vi "Save File Create Default File.vi"(7 "Type":enum16{"Pass Default", "Write Default"}(ring), 11 "Config Path":path) -> (3 "Default Configuration":string[][](array[string]))   [LabVIEW 2016, in "File Setup.lvlib"]
uses:
  File Setup.lvlib
  <vilib>/Utility/file.llb/Write To Spreadsheet File (string).vi
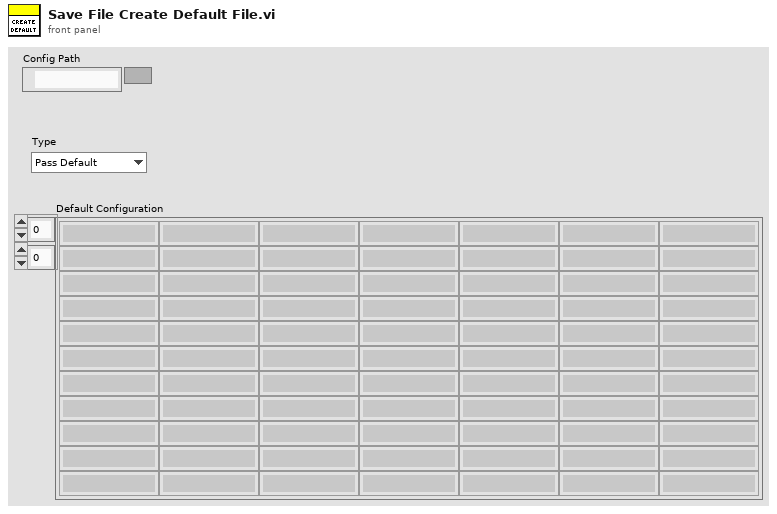
[diagram p1: front panel]
types:
  T1 = enum16{"open", "replace", "create", "open or create", "replace or create", "replace or create with confirmation"}
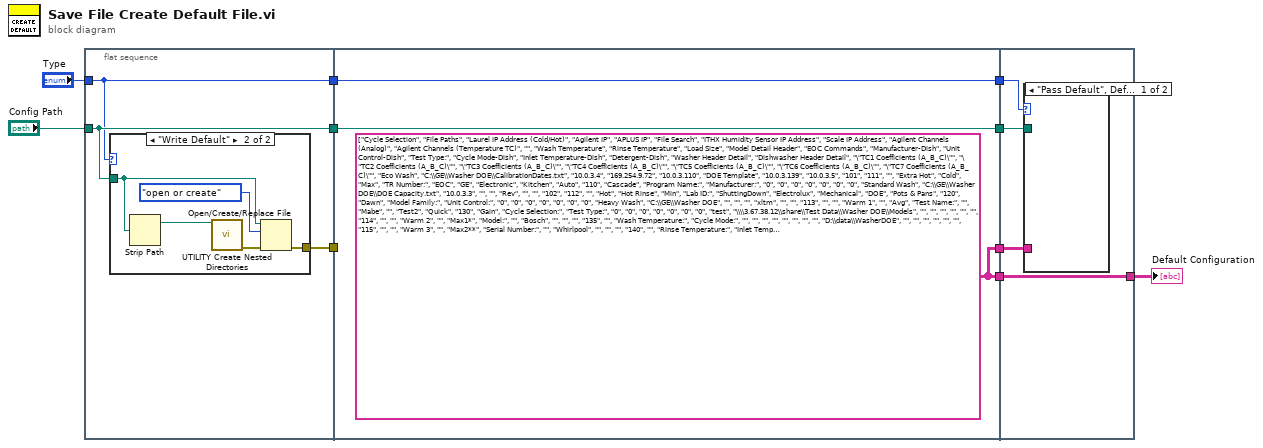
[diagram p0: block diagram]
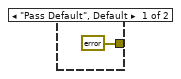
[diagram p2: hidden frame]
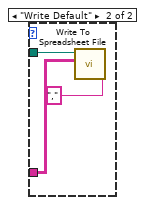
[diagram p3: hidden frame]
diagram:
  n1 = flat-sequence {
    tunnel: [w12] -> w10
    tunnel: [w13] -> w9
    tunnel: "Config Path" -> [w12]
    tunnel: "Type" -> [w11]
    tunnel: [w11] -> w1
    tunnel: w10 -> [w21]
    tunnel: w9 -> [_]
    tunnel: [w22] -> w6
    tunnel: [w22] -> w5
    tunnel: [w21] -> w4
    tunnel: [w20] -> w2
    tunnel: w1 -> [w20]
    tunnel: [w26] -> w7
    tunnel: w6 -> [w26]
    tunnel: w5 -> [w25]
    tunnel: w4 -> [w24]
    tunnel: w2 -> [w23]
    frame #0 {
      n2 = case shown="\"Write Default\"" w11 {
        tunnel: [errorcluster {"status"=FALSE, "code"=0, "source"=""} ("error out") w17] -> w13
        tunnel: w12 -> [_ w15]
        frame "Pass Default", Default {
        }
        frame "Write Default" {
          n3 = Strip Path(path=w15) -> (stripped path=w16:path)  [unwired: 1 out]
          n4 = call "UTILITY Create Nested Directories.vi"("path to create"=w16) -> ("error out"=w18:errorcluster)  [unwired: 12 in, 2 out]
          n5 = Open/Create/Replace File(file path (use dialog)=w15, error in=w18, operation (0:open)=T1."open or create") -> (error out=w17:errorcluster)  [unwired: 3 in, 2 out]
        }
      }
    }
    frame #1 {
      w22 = string[][] [["Cycle Selection", "File Paths", "Laurel IP Address (Cold/Hot)", "Agilent IP", "APLUS IP", "File Search", "ITHX Humidity Sensor IP Address", "Scale IP Address", "Agilent Channels (Analog)", "Agilent Channels (Temperature TC)", "", "Wash Temperature", "Rinse Temperature", "Load Size", "Model Detail Header", "EOC Commands", "Manufacturer-Dish", "Unit Control-Dish", "Test Type:", "Cycle Mode-Dish", "Inlet Temperature-Dish", "Detergent-Dish", "Washer Header Detail", "Dishwasher Header Detail", "\"TC1 Coefficients (A_B_C)\"", "\"TC2 Coefficients (A_B_C)\"", "\"TC3 Coefficients (A_B_C)\"", "\"TC4 Coefficients (A_B_C)\"", "\"TC5 Coefficients (A_B_C)\"", "\"TC6 Coefficients (A_B_C)\"", "\"TC7 Coefficients (A_B_C)\""], ["Eco Wash", "C:\\GE\\Washer DOE\\CalibrationDates.txt", "10.0.3.4", "169.254.9.72", "10.0.3.110", "DOE Template", "10.0.3.139", "10.0.3.5", "101", "111", "", "Extra Hot", "Cold", "Max", "TR Number:", "EOC", "GE", "Electronic", "Kitchen", "Auto", "110", "Cascade", "Program Name:", "Manufacturer:", "0", "0", "0", "0", "0", "0", "0"], ["Standard Wash", "C:\\GE\\Washer DOE\\DOE Capacity.txt", "10.0.3.3", "", "", "Rev", "", "", "102", "112", "", "Hot", "Hot Rinse", "Min", "Lab ID:", "ShuttingDown", "Electrolux", "Mechanical", "DOE", "Pots & Pans", "120", "Dawn", "Model Family:", "Unit Control:", "0", "0", "0", "0", "0", "0", "0"], ["Heavy Wash", "C:\\GE\\Washer DOE", "", "", "", "xltm", "", "", "113", "", "", "Warm 1", "", "Avg", "Test Name:", "", "Mabe", "", "Test2", "Quick", "130", "Gain", "Cycle Selection:", "Test Type:", "0", "0", "0", "0", "0", "0", "0"], ["test", "\\\\3.67.38.12\\share\\Test Data\\Washer DOE\\Models", "", "", "", "", "", "", "114", "", "", "Warm 2", "", "Max1*", "Model:", "", "Bosch", "", "", "", "135", "", "Wash Temperature:", "Cycle Mode:", "", "", "", "", "", "", ""], ["", "D:\\data\\WasherDOE", "", "", "", "", "", "", "115", "", "", "Warm 3", "", "Max2**", "Serial Number:", "", "Whirlpool", "", "", "", "140", "", "Rinse Temperature:", "Inlet Temperature (F):", "", "", "", "", "", "", ""], ["", "C:\\GE\\Washer DOE\\DOE_Backup.ini", "", "", "", "", "", "", "116", "", "", "Cold", "", "", "Station ID:", "", "", "", "", "", "", "", "Load Size:", "Detergent:", "", "", "", "", "", "", ""], ["", "", "", "", "", "", "", "", "", "", "", "Note ", "", "", "Engineer:", "", "", "", "", "", "", "", "Hot Water Temperature (Fahrenheit):", "Auto Cup Weight (gm):", "", "", "", "", "", "", ""], ["", "", "", "", "", "", "", "", "", "", "", "", "", "", "Technician", "", "", "", "", "", "", "", "Cold Water Temperature (Fahrenheit):", "Open Cup Weight (gm):", "", "", "", "", "", "", ""], ["", "", "", "", "", "", "", "", "", "", "", "", "", "", "Water Pressure:", "", "", "", "", "", "", "", "Capacity (cu.ft)", "", "", "", "", "", "", "", ""], ["", "", "", "", "", "", "", "", "", "", "", "", "", "", "Ambient RH:", "", "", "", "", "", "", "", "Initial Cloth Weight:", "", "", "", "", "", "", "", ""], ["", "", "", "", "", "", "", "", "", "", "", "", "", "", "Supply Voltage:", "", "", "", "", "", "", "", "Cloth Lot:", "", "", "", "", "", "", "", ""], ["", "", "", "", "", "", "", "", "", "", "", "", "", "", "Frequency:", "", "", "", "", "", "", "", "", "", "", "", "", "", "", "", ""], ["", "", "", "", "", "", "", "", "", "", "", "", "", "", "Build:", "", "", "", "", "", "", "", "", "", "", "", "", "", "", "", ""]] ("Calibration With Header 2")
    }
    frame #2 {
      n6 = case shown="\"Pass Default\", Default" w23 {
        tunnel: w25 -> [_ w29]
        tunnel: w24 -> [_ w28]
        frame "Pass Default", Default {
        }
        frame "Write Default" {
          n7 = call-poly <vilib>:"Write To Spreadsheet File.vi"("delimiter (\\t)"="," ("delimiter (\\t)"), "2D data"=w29, "file path (dialog if empty)"=w28) -> ()  [unwired: 5 in, 1 out]
        }
      }
    }
  }
  "Default Configuration" <- w7
